vi "wait.vi"(11 "String":string) -> ()   [LabVIEW 2015]
panel:
  out "Waiting":bool
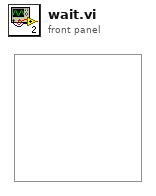
[diagram p1: front panel]
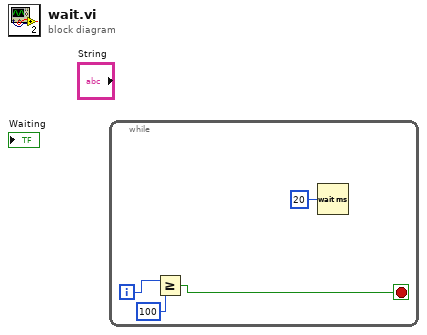
[diagram p0: block diagram]
diagram:
  n1 = while {
    i -> [w4]
    stop <- w2 stop-if-true
    n2 = Greater Or Equal?(x=w4, y=100 ("x")) -> (x >= y?=w2:bool)
    n3 = Wait (ms)(milliseconds to wait=u32 20) -> ()  [unwired: 1 out]
  }
